vi "StatRelRmsDeviation.vi"(3 "Array":dbl[](array[numeric])) -> (0 "Rel RMS Dev":dbl, 1 "Rel RMS Dev (%)":dbl)   [LabVIEW 2014]
uses:
  <vilib>/Analysis/NI_AALBase.lvlib
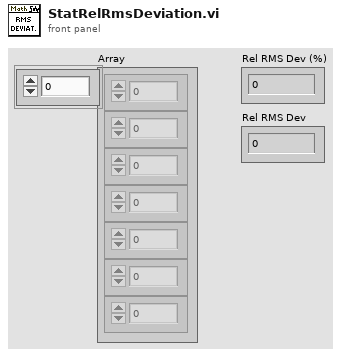
[diagram p1: front panel]
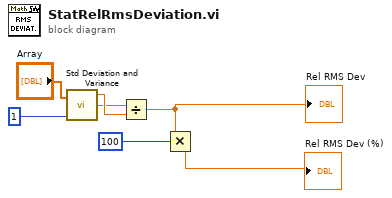
[diagram p0: block diagram]
diagram:
  n1 = call <vilib>:"Std Deviation and Variance.vi"("X"="Array", "Weighting (Sample)"=1) -> ("mean"=w2:dbl, "standard deviation"=w1:dbl)  [unwired: 1 out]
  n2 = Divide(x=w1, y=w2) -> (x/y=w3:dbl)
  "Rel RMS Dev" <- w3
  n3 = Multiply(x=w3, y=100) -> (x*y=→"Rel RMS Dev (%)":dbl)
